vi "Arm Movement Garret.vi"(10 "angle voltage":dbl=0.1 format="%#_13g", 11 "Buttons[1]":bool) -> ()   [LabVIEW 2015]
uses:
  <vilib>/Rock Robotics/Network Tables/NT Write String.vi
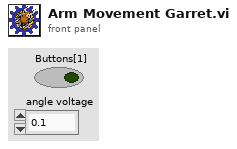
[diagram p1: front panel]
types:
  T1 = typedef "WPI_PotentiometerDevRef.ctl" = cluster{"DevStatus":errorcluster, "Analog Channel":T2, "Invert Output":bool}
  T2 = typedef "FPGA_AIChannel.ctl" = enum8{"AI 0", "AI 1", "AI 2", "AI 3", "AI MXP 0", "AI MXP 1", "AI MXP 2", "AI MXP 3", "Invalid"}
  T3 = typedef "WPI_EncoderDevRef.ctl" = cluster{"DevStatus":errorcluster, "EncoderIndex":T4, "CounterIndex":T5, "DistancePerCount":dbl, "Decoding Type":T6}
  T4 = typedef "FPGA_EncoderIdx.ctl" = enum8{"Enc 0", "Enc 1", "Enc 2", "Enc 3", "Enc 4", "Enc 5", "Enc 6", "Enc 7", "Invalid"}
  T5 = typedef "FPGA_CounterCtrSystemIndex.ctl" = enum8{"Ctr 0", "Ctr 1", "Ctr 2", "Ctr 3", "Ctr 4", "Ctr 5", "Ctr 6", "Ctr 7", "Invalid"}
  T6 = typedef "WPI_EncoderType.ctl" = enum16{"1x", "2x", "4x"}
  T7 = typedef "WPI_MotorControlDeviceRef.ctl" = cluster{"DeviceStatus":errorcluster, "Type":T8, "PWM":cluster{"PWM Channel":T9, "DeadBand":T10}, "CAN":cluster{"Device Number":u8, "Control Mode":T11, "Semaphore":T12, "Max Vout":dbl, "TalonSRX Control Mode":T13}, "Invert":bool}
  T8 = typedef "WPI_MotorControlType.ctl" = enum16{"PWM", "CAN", "CANTalonSRX"}
  T9 = typedef "FPGA_DIOPWMChannel.ctl" = enum8{"PWM 0", "PWM 1", "PWM 2", "PWM 3", "PWM 4", "PWM 5", "PWM 6", "PWM 7", "PWM 8", "PWM 9", "PWM MXP 0", "PWM MXP 1", "PWM MXP 2", "PWM MXP 3", "PWM MXP 4", "PWM MXP 5", "PWM MXP 6", "PWM MXP 7", "PWM MXP 8", "PWM MXP 9", "Invalid"}
  T10 = typedef "WPI_PWMDeadband.ctl" = cluster{"Name":string, "maxPositivePwm":i32, "minPositivePwm":i32, "centerPwm":i32, "maxNegativePwm":i32, "minNegativePwm":i32, "angularRange":u16}
  T11 = typedef "WPI_CANJaguar_ControlMode.ctl" = enum8{"Percent VBus", "Current", "Speed", "Position", "Voltage"}
  T12 = typedef "Semaphore RefNum" = refnum<k1>
  T13 = typedef "WPI_CANTalonSRX_APIControlMode.ctl" = enum8{"Percent VBus", "Speed", "Position", "Slave", "Unchanged / Invalid", "Voltage Compensation", "Current", "Motion Profile"}
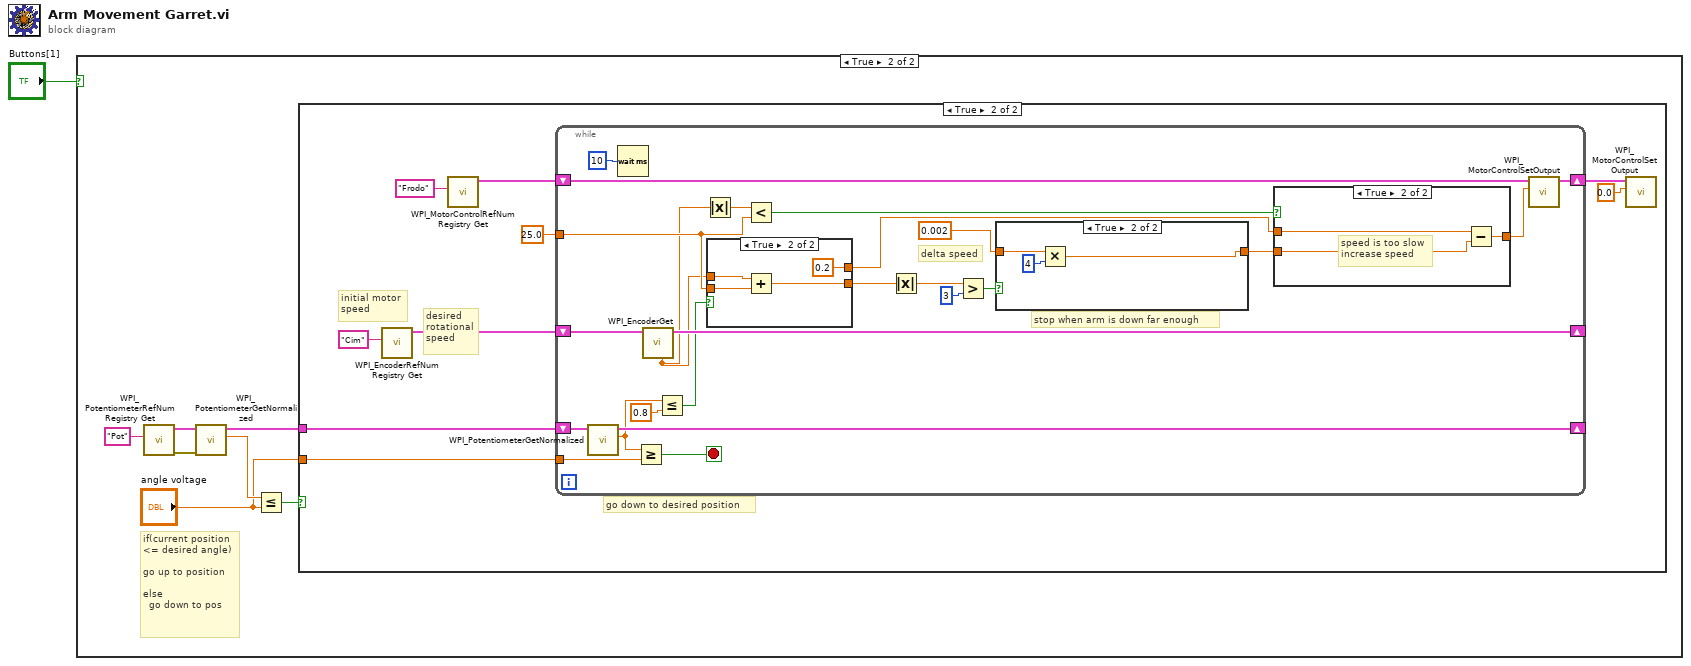
[diagram p0: block diagram]
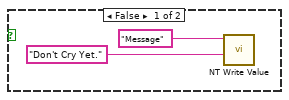
[diagram p2: hidden frame]
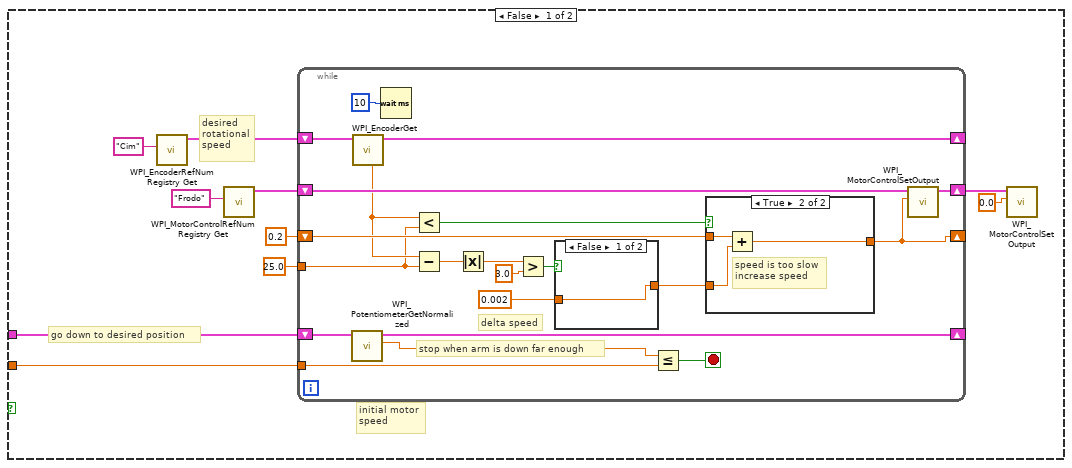
[diagram p3: hidden frame]
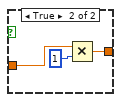
[diagram p4: hidden frame]
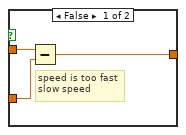
[diagram p5: hidden frame]
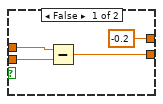
[diagram p6: hidden frame]
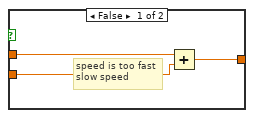
[diagram p8: hidden frame]
diagram:
  n1 = case shown="True" "Buttons[1]" {
    frame False {
      n2 = call-poly <vilib>:"NT Write Value.vi"("String"="Don't Cry Yet.", "Name"="Message") -> ()  [unwired: 9 in, 1 out]
    }
    frame True {
      # "if(current position\n<= desired angle)\n\ngo up to position\n\nelse\n  go down to pos"
      n3 = call <vilib>:"WPI_PotentiometerRefNum Registry Get.vi"("refnum name"="Pot") -> ("error out"=w8:errorcluster, "PotDevRef"=w9:T1)  [unwired: 9 in]
      n4 = call <vilib>:"WPI_PotentiometerGetNormalized.vi"("error in"=w8, "PotDevRef"=w9) -> ("Normalized Value"=w7:dbl, "PotDevRef"=w5:T1)  [unwired: 7 in, 1 out]
      n5 = Less Or Equal?(x=w7, y="angle voltage") -> (x <= y?=w6:bool)
      n6 = case shown="True" w6 {
        tunnel: w5 -> [w18 w53]
        tunnel: "angle voltage" -> [w17 w52]
        frame False {
          # "desired\nrotational\nspeed"
          # "initial motor\nspeed"
          # "go down to desired position"
          n7 = call <vilib>:"WPI_EncoderRefNum Registry Get.vi"("refnum name"="Cim") -> ("EncoderDevRef"=w12:T3)  [unwired: 9 in, 1 out]
          n8 = call <vilib>:"WPI_MotorControlRefNum Registry Get.vi"("refnum name"="Frodo") -> ("MotorControlDevRef"=w15:T7)  [unwired: 9 in, 1 out]
          n9 = while {
            shift-right: [w38] -> _
            shift-left: w18 -> [w41]
            shift-right: [w35] -> w20
            shift-left: w15 -> [w36]
            tunnel: w17 -> [w37]
            shift-right: [w32] -> _
            shift-left: 0.2 ("Output") -> [w33]
            tunnel: 25.0 ("y") -> [w27]
            shift-right: [w29] -> _
            shift-left: w12 -> [w30]
            stop <- w39 stop-if-true
            # "delta speed"
            # "stop when arm is down far enough"
            n10 = call <vilib>:"WPI_PotentiometerGetNormalized.vi"("PotDevRef"=w41) -> ("Normalized Value"=w40:dbl, "PotDevRef"=w38:T1)  [unwired: 8 in, 1 out]
            n11 = call <vilib>:"WPI_EncoderGet.vi"("EncoderDevRef"=w30) -> ("EncoderDevRef"=w29:T3, "Rate"=w28:dbl)  [unwired: 5 in, 4 out]
            n12 = Wait (ms)(milliseconds to wait=u32 10) -> ()  [unwired: 1 out]
            n13 = Less?(x=w28, y=w27) -> (x < y?=w34:bool)
            n14 = Subtract(x=w28, y=w27) -> (x-y=w26:dbl)
            n15 = Absolute Value(x=w26) -> (abs(x)=w25:dbl)
            n16 = Greater?(x=w25, y=3.0) -> (0:w23:bool)
            n17 = case shown="False" w23 {
              tunnel: 0.002 ("y") -> [w42 w45]
              tunnel: [w42 w43] -> w21
              frame False {
              }
              frame True {
                n18 = Multiply(x=w45, y=1) -> (x*y=w43:dbl)
              }
            }
            n19 = Less Or Equal?(x=w40, y=w37) -> (x <= y?=w39:bool)
            n20 = case shown="True" w34 {
              tunnel: w33 -> [w48 w51]
              tunnel: [w46 w50] -> w32
              tunnel: w21 -> [w47 w49]
              frame False {
                # "speed is too fast\nslow speed"
                n21 = Subtract(x=w48, y=w47) -> (x-y=w46:dbl)
              }
              frame True {
                # "speed is too slow\nincrease speed"
                n22 = Add(x=w51, y=w49) -> (x+y=w50:dbl)
              }
            }
            n23 = call <vilib>:"WPI_MotorControlSetOutput.vi"("Output"=w32, "MotorControlDevRef"=w36) -> ("MotorControlDevRef"=w35:T7)  [unwired: 7 in, 2 out]
          }
          n24 = call <vilib>:"WPI_MotorControlSetOutput.vi"("Output"=0.0, "MotorControlDevRef"=w20) -> ()  [unwired: 7 in, 3 out]
        }
        frame True {
          # "desired\nrotational\nspeed"
          # "initial motor\nspeed"
          # "go down to desired position"
          n25 = call <vilib>:"WPI_EncoderRefNum Registry Get.vi"("refnum name"="Cim") -> ("EncoderDevRef"=w55:T3)  [unwired: 9 in, 1 out]
          n26 = call <vilib>:"WPI_MotorControlRefNum Registry Get.vi"("refnum name"="Frodo") -> ("MotorControlDevRef"=w57:T7)  [unwired: 9 in, 1 out]
          n27 = while {
            shift-right: [w82] -> _
            shift-left: w53 -> [w84]
            shift-right: [w79] -> w60
            shift-left: w57 -> [w80]
            tunnel: w52 -> [w81]
            tunnel: 25.0 ("y") -> [w64]
            shift-right: [w74] -> _
            shift-left: w55 -> [w75]
            stop <- w83 stop-if-true
            # "delta speed"
            # "stop when arm is down far enough"
            n28 = call <vilib>:"WPI_PotentiometerGetNormalized.vi"("PotDevRef"=w84) -> ("Normalized Value"=w68:dbl, "PotDevRef"=w82:T1)  [unwired: 8 in, 1 out]
            n29 = Wait (ms)(milliseconds to wait=u32 10) -> ()  [unwired: 1 out]
            n30 = Greater Or Equal?(x=w68, y=w81) -> (x >= y?=w83:bool)
            n31 = call <vilib>:"WPI_EncoderGet.vi"("EncoderDevRef"=w75) -> ("EncoderDevRef"=w74:T3, "Rate"=w61:dbl)  [unwired: 5 in, 4 out]
            n32 = Less Or Equal?(x=w68, y=0.8) -> (x <= y?=w66:bool)
            n33 = Absolute Value(x=w61) -> (abs(x)=w62:dbl)
            n34 = case shown="True" w66 {
              tunnel: [-0.2 0.2] -> w65
              tunnel: w61 -> [w87 w91]
              tunnel: w64 -> [w86 w90]
              tunnel: [w85 w89] -> w63
              frame False {
                n35 = Subtract(x=w87, y=w86) -> (x-y=w85:dbl)
              }
              frame True {
                n36 = Add(x=w91, y=w90) -> (x+y=w89:dbl)
              }
            }
            n37 = Less?(x=w62, y=w64) -> (x < y?=w78:bool)
            n38 = Absolute Value(x=w63) -> (abs(x)=w73:dbl)
            n39 = Greater?(x=w73, y=3) -> (0:w71:bool)
            n40 = case shown="True" w71 {
              tunnel: 0.002 ("y") -> [w93 w96]
              tunnel: [w93 w94] -> w69
              frame False {
              }
              frame True {
                n41 = Multiply(x=w96, y=4) -> (x*y=w94:dbl)
              }
            }
            n42 = case shown="True" w78 {
              tunnel: w65 -> [w99 w102]
              tunnel: [w97 w101] -> w77
              tunnel: w69 -> [w98 w100]
              frame False {
                # "speed is too fast\nslow speed"
                n43 = Add(x=w99, y=w98) -> (x+y=w97:dbl)
              }
              frame True {
                # "speed is too slow\nincrease speed"
                n44 = Subtract(x=w102, y=w100) -> (x-y=w101:dbl)
              }
            }
            n45 = call <vilib>:"WPI_MotorControlSetOutput.vi"("Output"=w77, "MotorControlDevRef"=w80) -> ("MotorControlDevRef"=w79:T7)  [unwired: 7 in, 2 out]
          }
          n46 = call <vilib>:"WPI_MotorControlSetOutput.vi"("Output"=0.0, "MotorControlDevRef"=w60) -> ()  [unwired: 7 in, 3 out]
        }
      }
    }
  }
